vi "Main.vi"() -> ()   [LabVIEW 2011]
doc: "Use this template to build a simple state machine design pattern. Each state executes code and determines which state to transition to."
uses:
  controls/Data.ctl
  controls/State.ctl
panel:
  in  "Feeder Input":i16=1
  in  "Corridor Input":i16=2
  out "refnum out":refnum<k1>
  in  "Feeder Delay":u32=500
  in  "Corridor Delay":u32=500
  in  "Sample Delay":i32=50
  out "Data":T1
  out "Beam":u32
  in  "@Feeder":bool
  in  "Feeder Enable":bool
  in  "EoCo":bool
  in  "Exit":bool
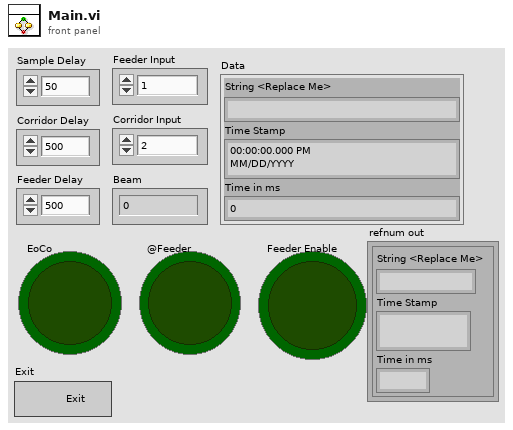
[diagram p1: front panel]
types:
  T1 = typedef "Data.ctl" = cluster{"String <Replace Me>":string, "Time Stamp":timestamp, "Time in ms":dbl}
  T2 = typedef "State.ctl" = enum16{"Initialize", "Refresh", "Wait for Event", "End of Corridor", "End of Corridor Delay", "Feed", "Feed Delay", "Exit"}
  T3 = enum16{"open", "replace", "create", "open or create", "replace or create", "replace or create with confirmation"}
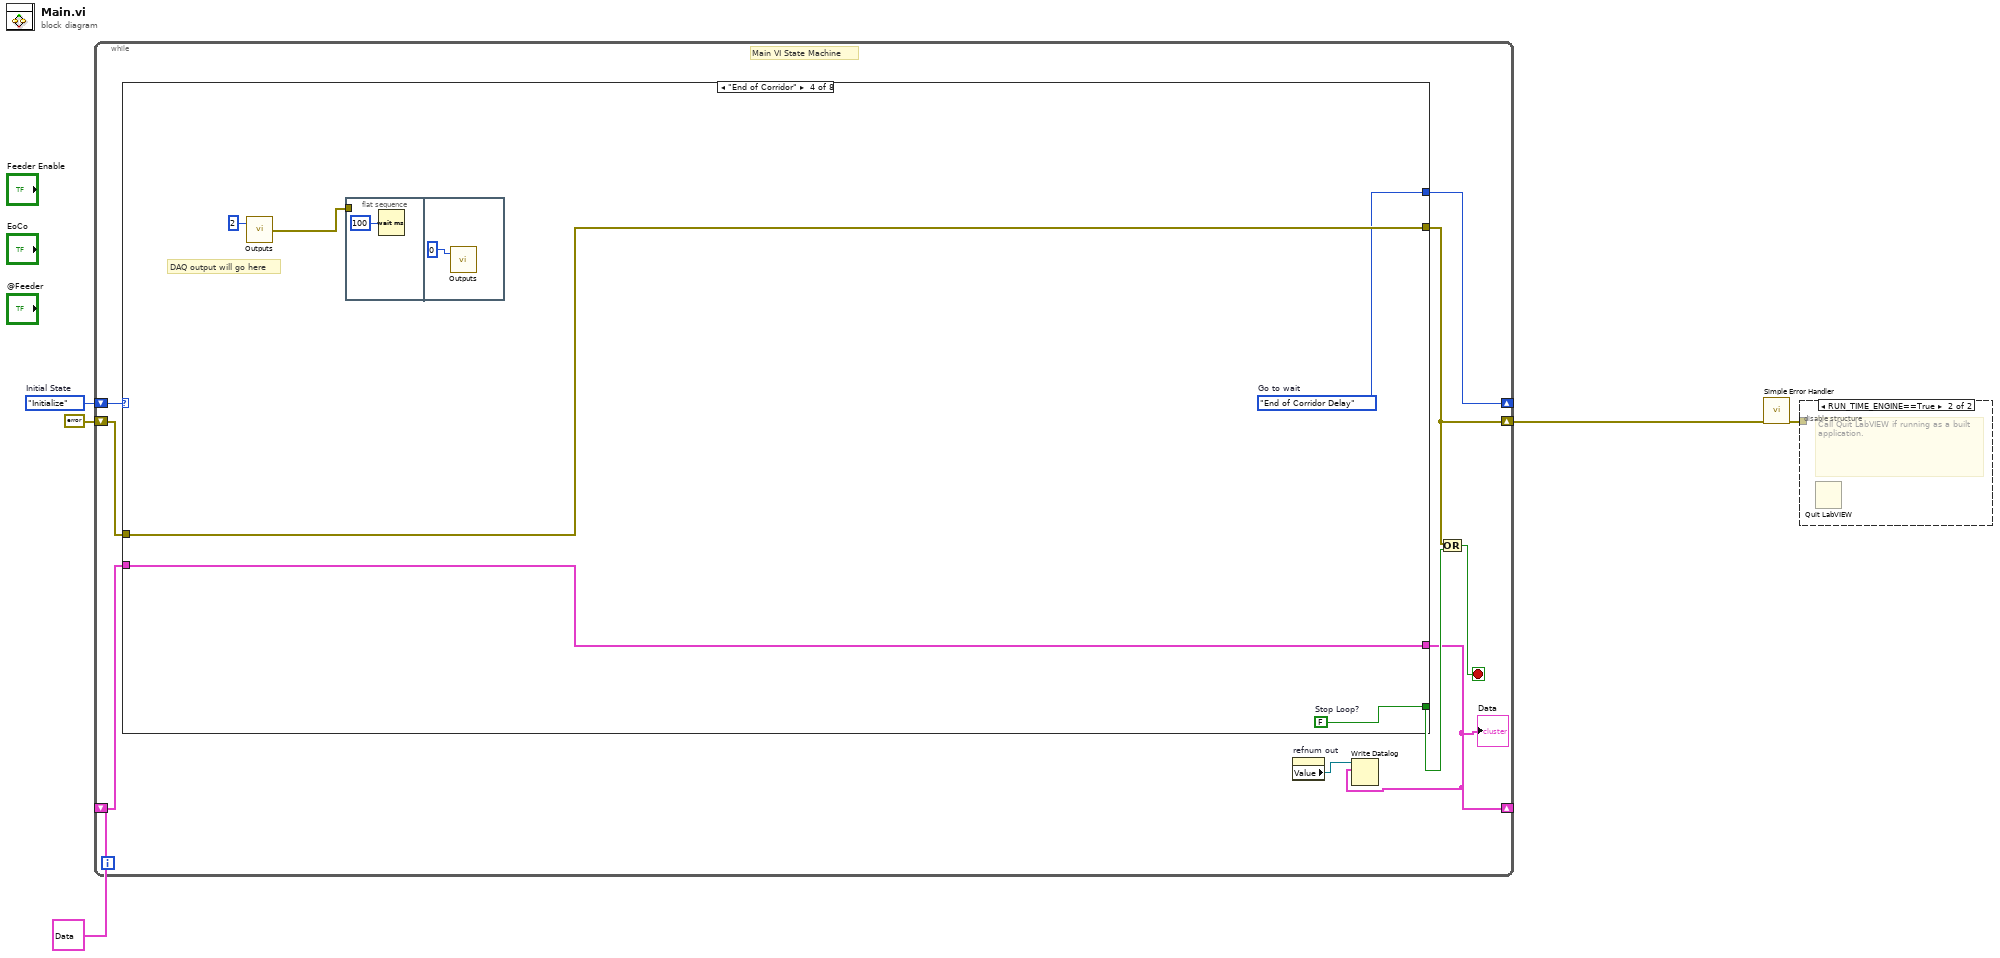
[diagram p0: block diagram]
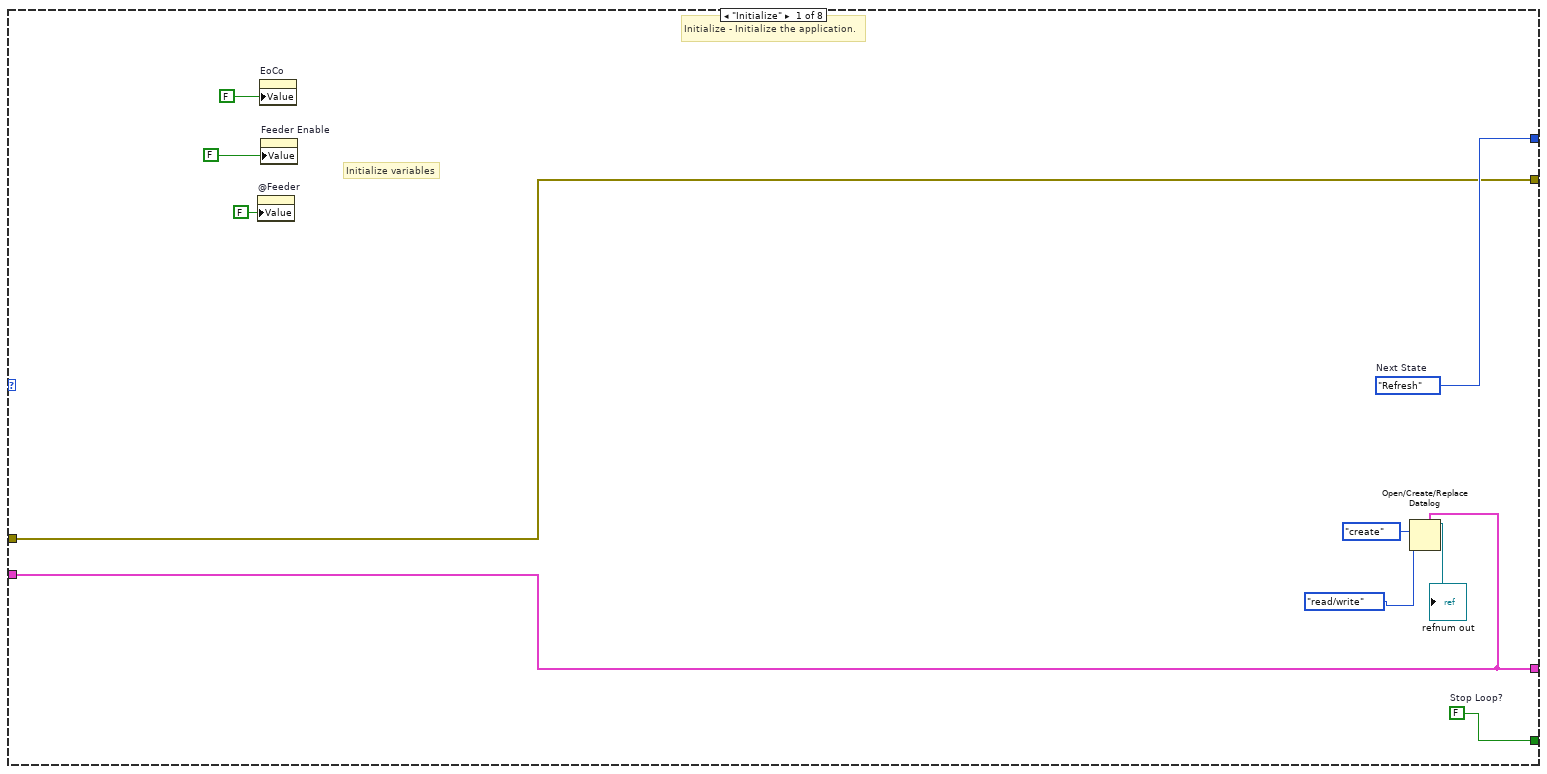
[diagram p3: hidden frame]
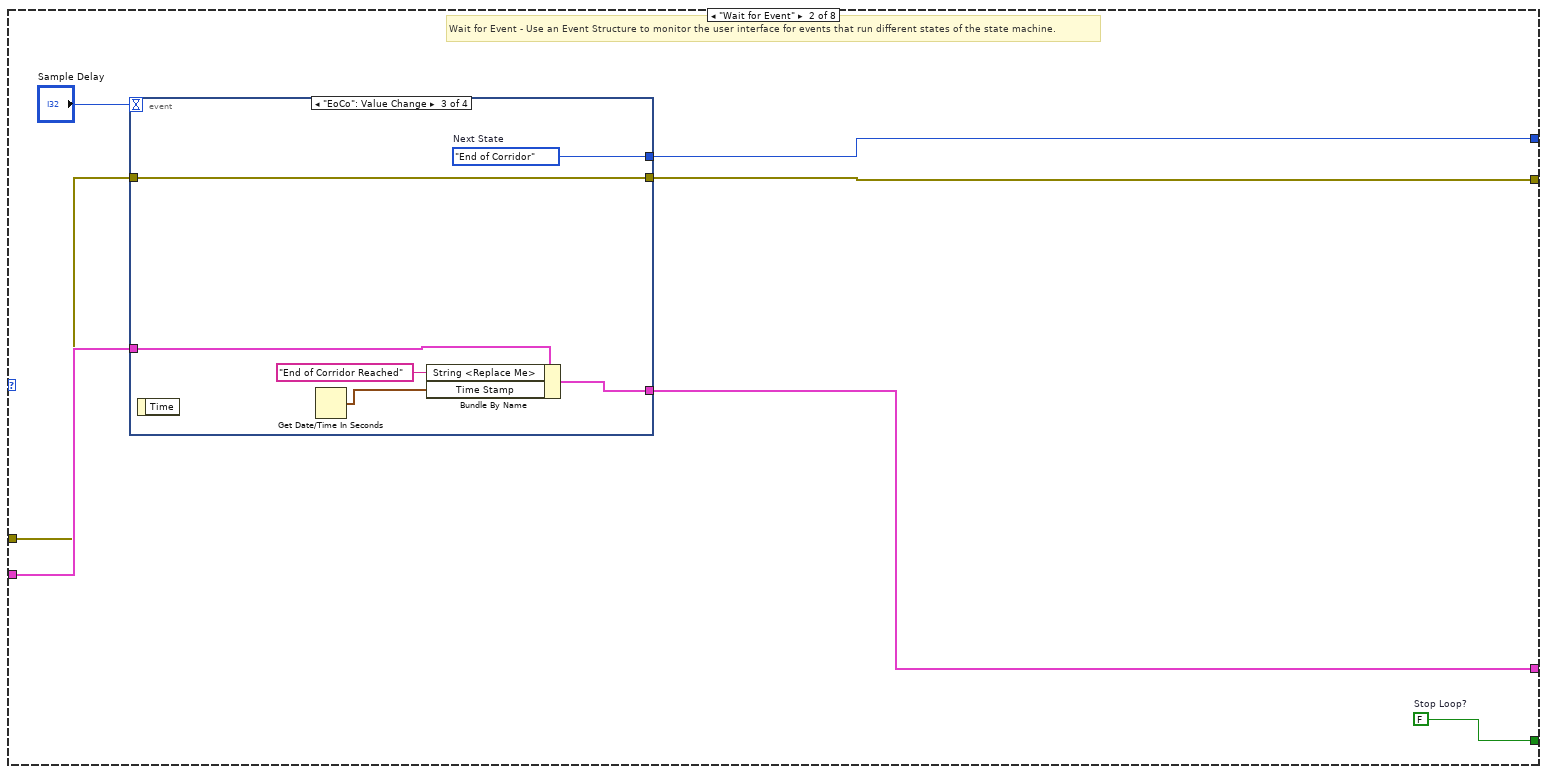
[diagram p4: hidden frame]
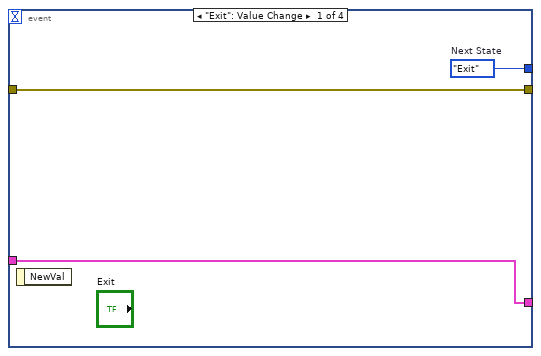
[diagram p5: hidden frame]
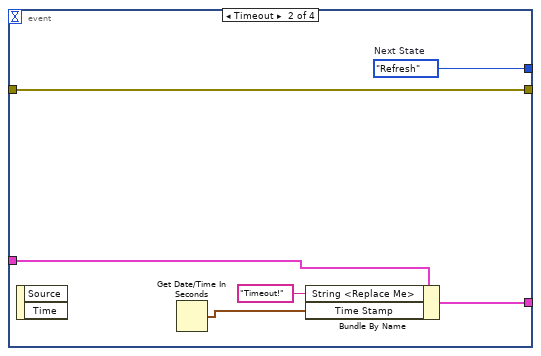
[diagram p6: hidden frame]
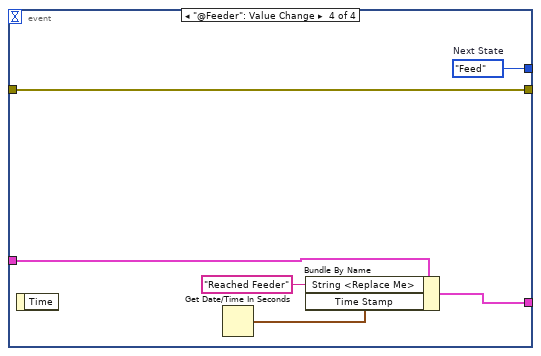
[diagram p7: hidden frame]
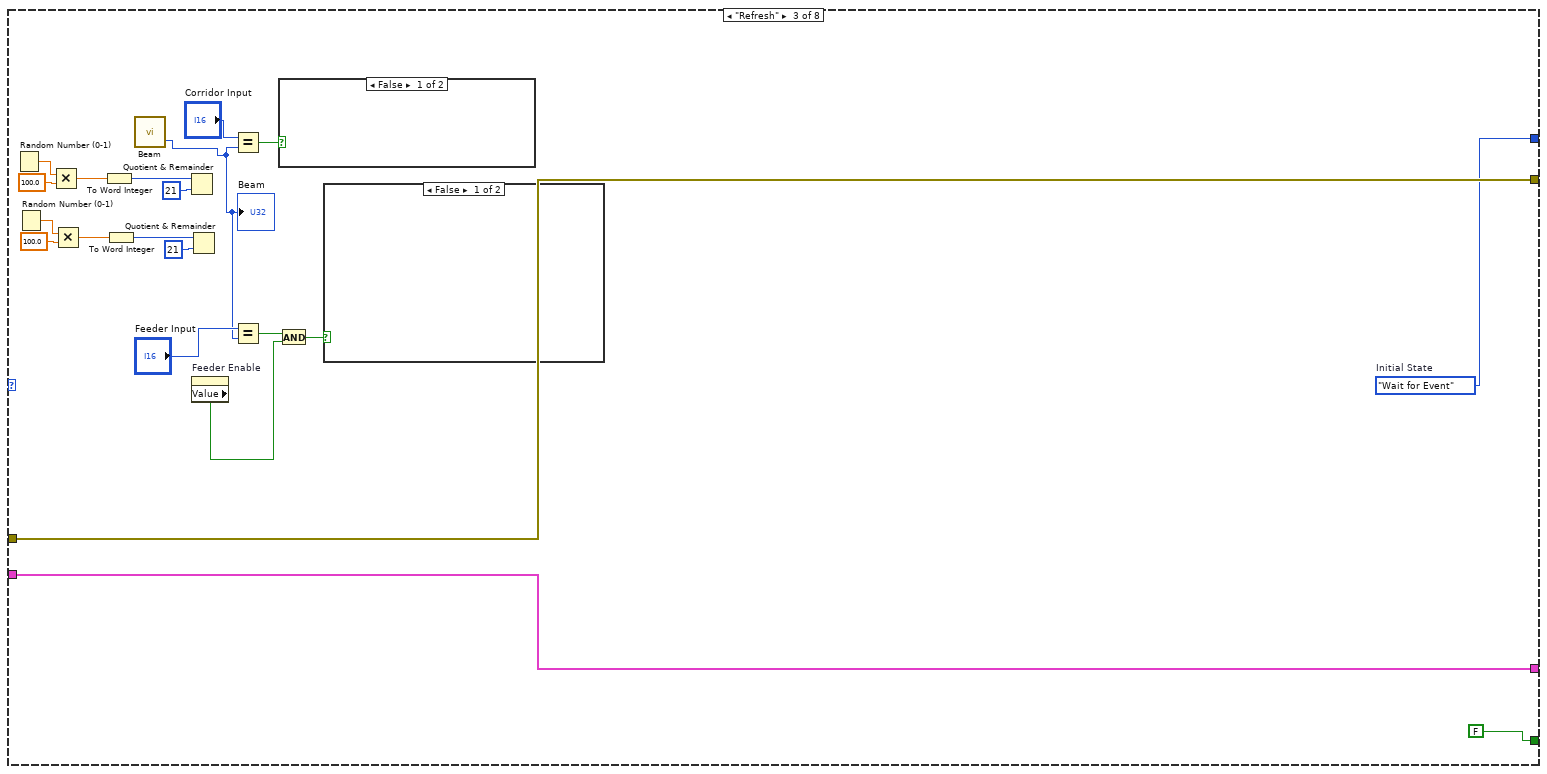
[diagram p8: hidden frame]
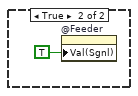
[diagram p9: hidden frame]
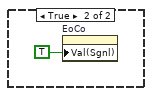
[diagram p10: hidden frame]
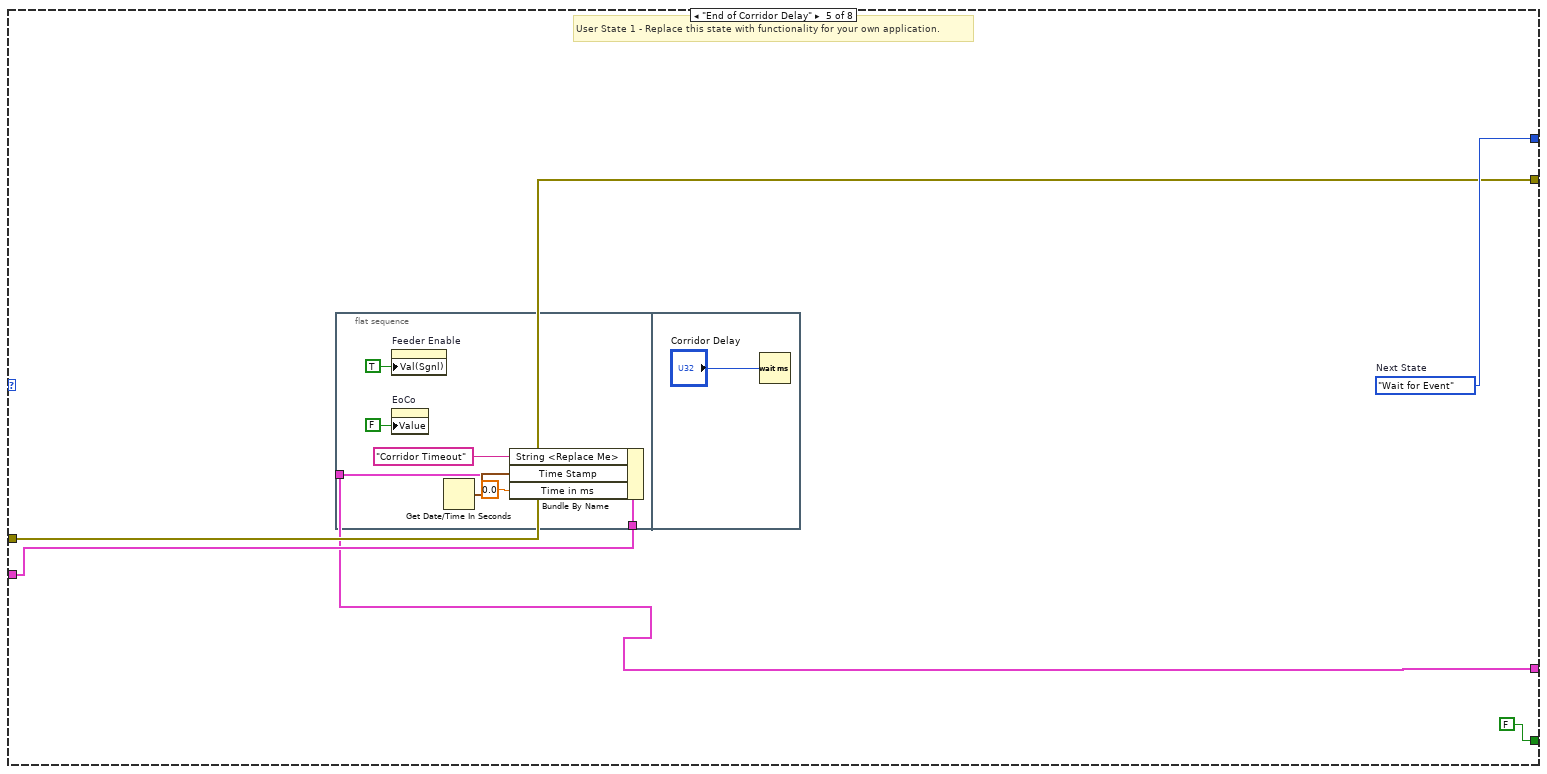
[diagram p11: hidden frame]
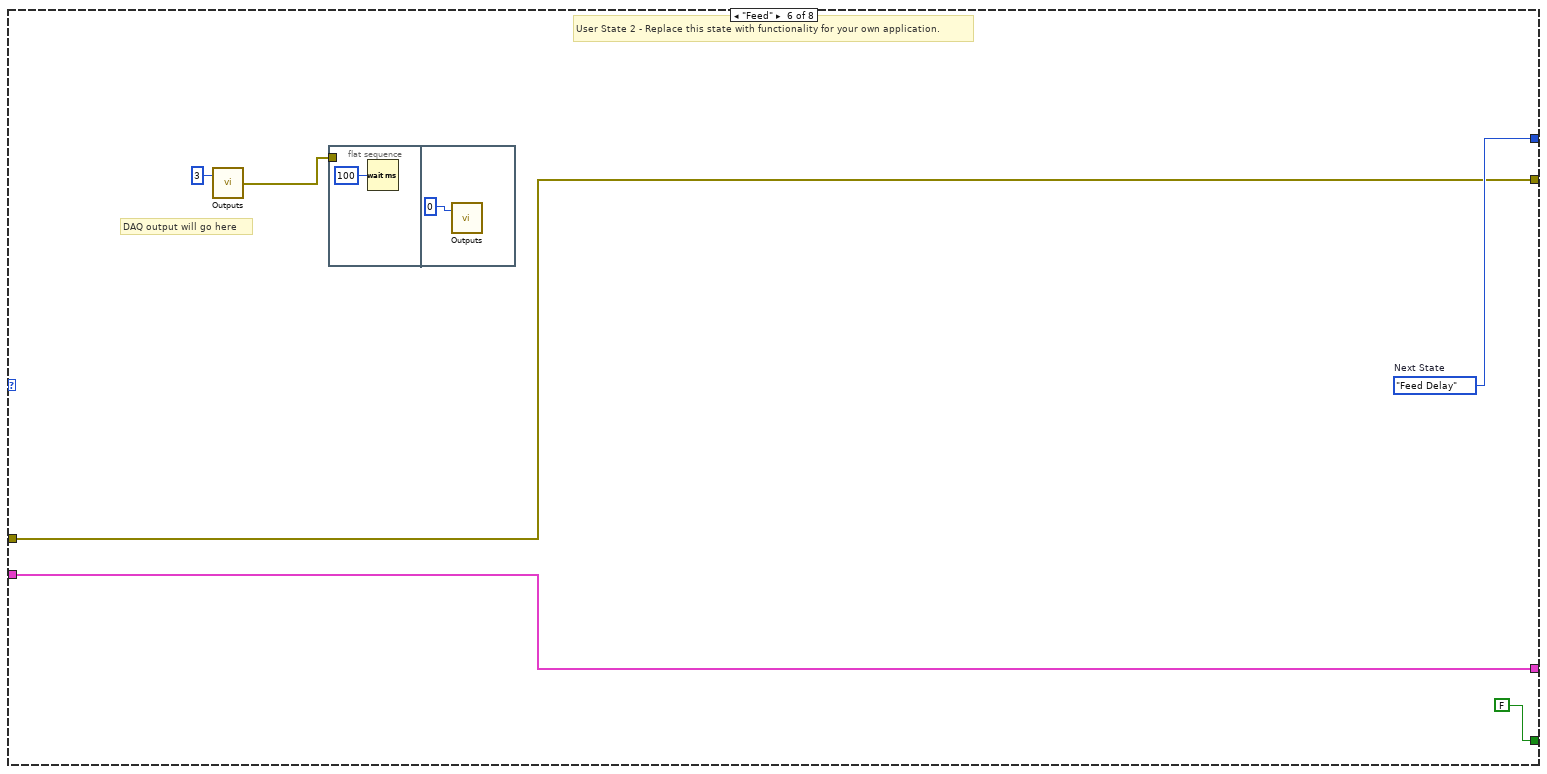
[diagram p12: hidden frame]
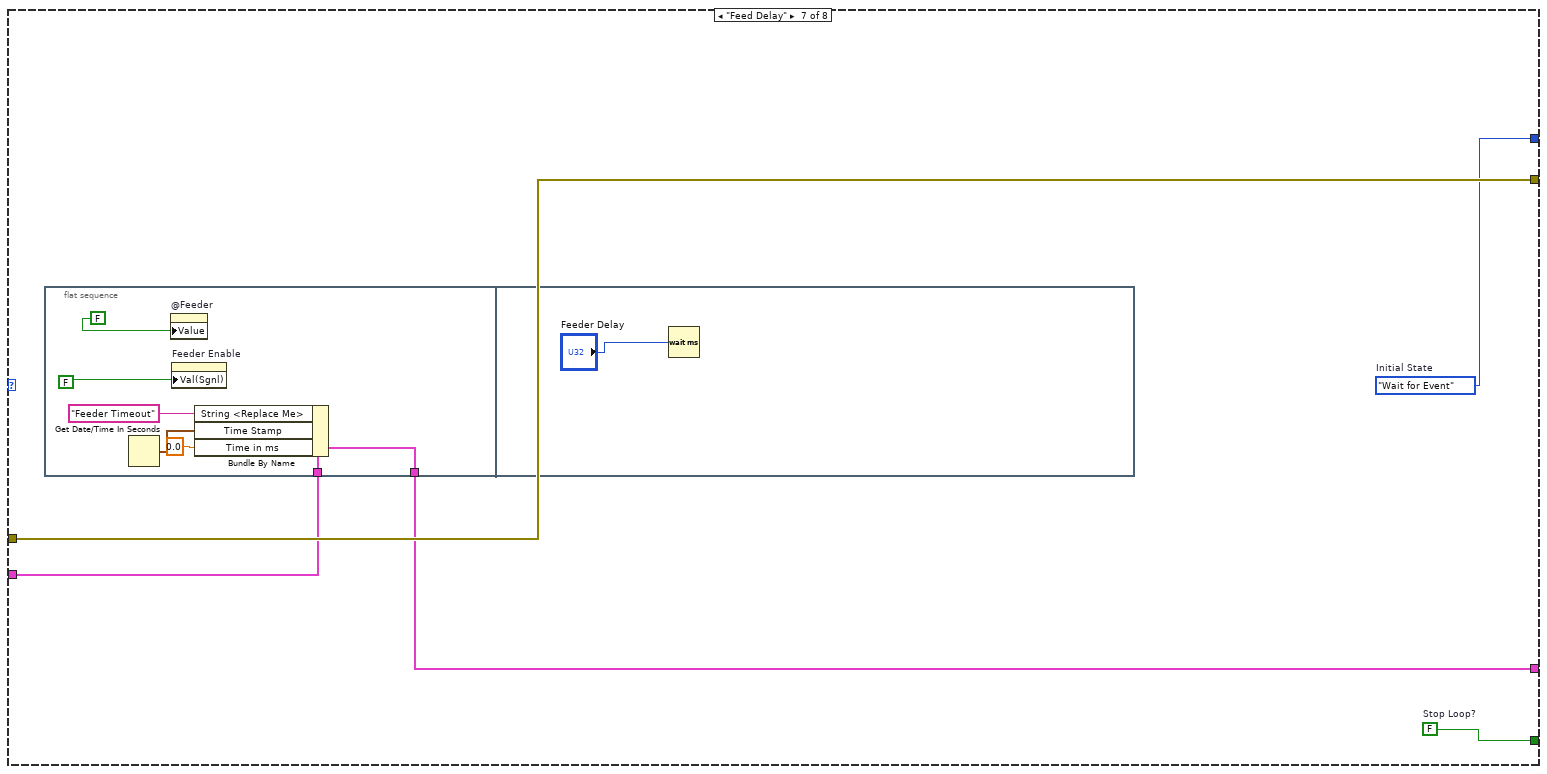
[diagram p13: hidden frame]
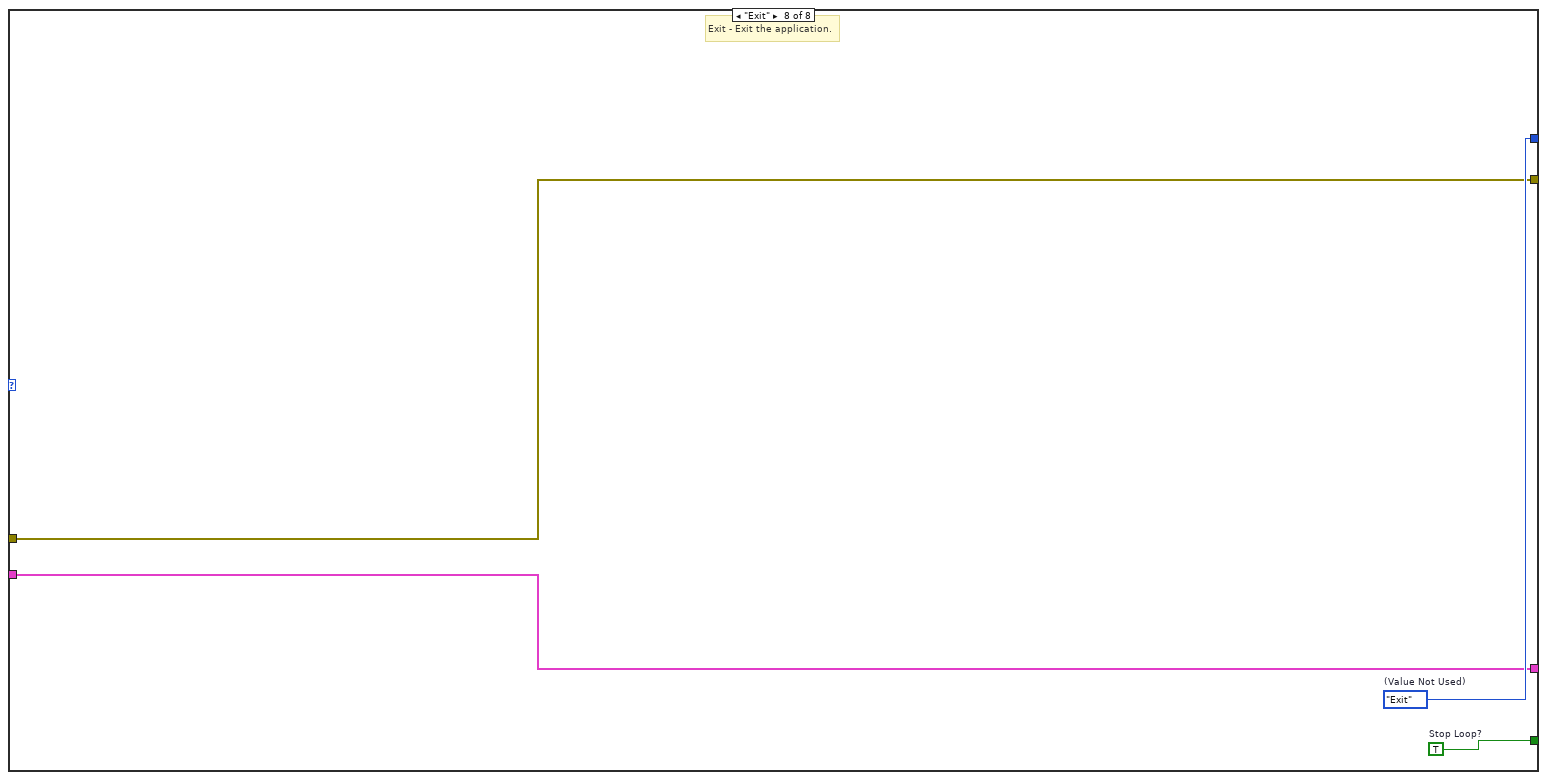
[diagram p14: hidden frame]
diagram:
  w5 = State."Initialize"  # Initial State
  n1 = while {
    shift-right: [w13] -> _
    shift-left: w5 -> [w14]
    shift-right: [w7] -> _
    shift-left: T1 {"String <Replace Me>"="", "Time Stamp"=timestamp(0 s since 1904-01-01), "Time in ms"=0.0} ("Data") -> [w12]
    shift-right: [w8] -> w2
    shift-left: errorcluster {"status"=FALSE, "code"=0, "source"=""} ("error constant") -> [w11]
    stop <- w9 stop-if-true
    # "Main VI State Machine"
    n2 = case shown="\"End of Corridor\"" w14 {
      tunnel: [w24 w31 w71 w79 w88 w102 w108 w121] -> w13
      tunnel: [w23 w30 FALSE ("Stop Loop?") w78 FALSE ("Stop Loop?") FALSE ("Stop Loop?") w107 w118] -> w10
      tunnel: w12 -> [w16 w29 w73 w81 w85 w100 w106 w120]
      tunnel: [w16 w28 w73 w81 w84 w100 w105 w120] -> w7
      tunnel: w11 -> [w22 w27 w72 w80 w86 w99 w109 w119]
      tunnel: [w22 w26 w72 w80 w86 w99 w109 w119] -> w8
      frame "Initialize" {
        w23 = FALSE  # Stop Loop?
        w24 = State."Refresh"  # Next State
        # "Initialize variables"
        # "Initialize - Initialize the application."
        n3 = property on="@Feeder" class="Bool (strict)"("Value"=FALSE ("@Feeder")) -> ()  [unwired: 2 in, 2 out]
        n4 = property on="EoCo" class="Bool (strict)"("Value"=FALSE ("Value (Signaling)")) -> ()  [unwired: 2 in, 2 out]
        n5 = property on="Feeder Enable" class="Bool (strict)"("Value"=FALSE) -> ()  [unwired: 2 in, 2 out]
        n6 = Open/Create/Replace Datalog(5:w16, 9:enum16{"read/write", "read-only", "write-only"}."read/write" ("access (0:read/write)"), 10:T3."create" ("operation (0:open)")) -> (3:→"refnum out":refnum<k1>)  [unwired: 3 in, 2 out]
      }
      frame "Wait for Event" {
        w30 = FALSE  # Stop Loop?
        # "Wait for Event - Use an Event Structure to monitor the user interface for events that run different states of the state machine."
        n7 = event shown="[2] \"EoCo\": Value Change" {
          selector: _ -> [_ _ _ _]
          dyn-events: _ -> [_ _ _ _]
          timeout: "Sample Delay" -> [_ _ _ _]
          tunnel: [w34 w39 w46 w52] -> w31
          tunnel: w29 -> [w33 w36 w45 w51]
          tunnel: [w33 w38 w44 w50] -> w28
          tunnel: w27 -> [w32 w40 w42 w48]
          tunnel: [w32 w40 w42 w48] -> w26
          event "Exit": Value Change {
            w34 = State."Exit"  # Next State
            n8 = event-data() -> ()  [unwired: 1 in, 1 out]
          }
          event Timeout {
            w39 = State."Refresh"  # Next State
            n9 = event-data() -> ()  [unwired: 1 in, 2 out]
            n10 = Get Date/Time In Seconds() -> (seconds since 1Jan1904=w35:timestamp)
            n11 = Bundle By Name(cluster=w36, "String <Replace Me>"="Timeout!", "Time Stamp"=w35) -> (w38:T1)
          }
          event "EoCo": Value Change {
            w46 = State."End of Corridor"  # Next State
            n12 = event-data() -> ()  [unwired: 1 in, 1 out]
            n13 = Get Date/Time In Seconds() -> (seconds since 1Jan1904=w41:timestamp)
            n14 = Bundle By Name(cluster=w45, "String <Replace Me>"="End of Corridor Reached" ("Running User State 1"), "Time Stamp"=w41) -> (w44:T1)
          }
          event "@Feeder": Value Change {
            w52 = State."Feed"  # Next State
            n15 = event-data() -> ()  [unwired: 1 in, 1 out]
            n16 = Get Date/Time In Seconds() -> (seconds since 1Jan1904=w47:timestamp)
            n17 = Bundle By Name(cluster=w51, "String <Replace Me>"="Reached Feeder" ("Running User State 2"), "Time Stamp"=w47) -> (w50:T1)
          }
        }
      }
      frame "Refresh" {
        w71 = State."Wait for Event"  # Initial State
        n18 = Random Number (0-1)() -> (number: 0 to 1=w59:dbl)
        n19 = Random Number (0-1)() -> (number: 0 to 1=w66:dbl)
        n20 = Multiply(x=w59, y=100.0) -> (x*y=w60:dbl)
        n21 = Multiply(x=w66, y=100.0) -> (x*y=w65:dbl)
        n22 = To Word Integer(number=w60) -> (16bit integer=w61:i16)
        n23 = To Word Integer(number=w65) -> (16bit integer=w68:i16)
        n24 = call "Beam.vi"() -> ("return type"=w53:i16)  [unwired: 1 in, 1 out]
        "Beam" <- w53
        n25 = Quotient & Remainder(x=w61, y=u32 21) -> ()  [unwired: 2 out]
        n26 = Quotient & Remainder(x=w68, y=i16 21) -> ()  [unwired: 2 out]
        n27 = property on="Feeder Enable" class="Bool (strict)"() -> ("Value"=w70:bool)  [unwired: 2 in, 2 out]
        n28 = Equal?(x="Corridor Input", y=w53) -> (x = y?=w62:bool)
        n29 = Equal?(x="Feeder Input", y=w53) -> (x = y?=w63:bool)
        n30 = case shown="False" w62 {
          frame False {
          }
          frame True {
            n31 = property on="EoCo" class="Bool (strict)"("Val(Sgnl)"=TRUE ("Value (Signaling)")) -> ()  [unwired: 2 in, 2 out]
          }
        }
        n32 = And(x=w63, y=w70) -> (x .and. y?=w64:bool)
        n33 = case shown="False" w64 {
          frame False {
          }
          frame True {
            n34 = property on="@Feeder" class="Bool (strict)"("Val(Sgnl)"=TRUE ("Value (Signaling)")) -> ()  [unwired: 2 in, 2 out]
          }
        }
      }
      frame "End of Corridor" {
        w78 = FALSE  # Stop Loop?
        w79 = State."End of Corridor Delay"  # Go to wait
        # "DAQ output will go here"
        n35 = call "Outputs.vi"("Value"=i16 2) -> ("error out"=w77:errorcluster)  [unwired: 1 in]
        n36 = flat-sequence {
          tunnel: w77 -> [_]
          frame #0 {
            n37 = Wait (ms)(milliseconds to wait=u32 100) -> ()  [unwired: 1 out]
          }
          frame #1 {
            n38 = call "Outputs.vi"("Value"=i16 0) -> ()  [unwired: 1 in, 1 out]
          }
        }
      }
      frame "End of Corridor Delay" {
        w88 = State."Wait for Event"  # Next State
        # "User State 1 - Replace this state with functionality for your own application."
        n39 = flat-sequence {
          tunnel: w85 -> [w90]
          tunnel: [w89] -> w84
          frame #0 {
            n40 = property on="Feeder Enable" class="Bool (strict)"("Val(Sgnl)"=TRUE ("Value (Signaling)")) -> ()  [unwired: 2 in, 2 out]
            n41 = property on="EoCo" class="Bool (strict)"("Value"=FALSE ("Value (Signaling)")) -> ()  [unwired: 2 in, 2 out]
            n42 = Get Date/Time In Seconds() -> (seconds since 1Jan1904=w92:timestamp)
            n43 = Bundle By Name(cluster=w90, "String <Replace Me>"="Corridor Timeout", "Time Stamp"=w92, "Time in ms"=0.0) -> (w89:T1)
          }
          frame #1 {
            n44 = Wait (ms)(milliseconds to wait="Corridor Delay") -> ()  [unwired: 1 out]
          }
        }
      }
      frame "Feed" {
        w102 = State."Feed Delay"  # Next State
        # "DAQ output will go here"
        # "User State 2 - Replace this state with functionality for your own application."
        n45 = call "Outputs.vi"("Value"=i16 3) -> ("error out"=w98:errorcluster)  [unwired: 1 in]
        n46 = flat-sequence {
          tunnel: w98 -> [_]
          frame #0 {
            n47 = Wait (ms)(milliseconds to wait=u32 100) -> ()  [unwired: 1 out]
          }
          frame #1 {
            n48 = call "Outputs.vi"("Value"=i16 0) -> ()  [unwired: 1 in, 1 out]
          }
        }
      }
      frame "Feed Delay" {
        w107 = FALSE  # Stop Loop?
        w108 = State."Wait for Event"  # Initial State
        n49 = flat-sequence {
          tunnel: w106 -> [w111]
          tunnel: [w110] -> w105
          frame #0 {
            n50 = Get Date/Time In Seconds() -> (seconds since 1Jan1904=w113:timestamp)
            n51 = property on="@Feeder" class="Bool (strict)"("Value"=FALSE ("@Feeder")) -> ()  [unwired: 2 in, 2 out]
            n52 = property on="Feeder Enable" class="Bool (strict)"("Val(Sgnl)"=FALSE ("Value (Signaling)")) -> ()  [unwired: 2 in, 2 out]
            n53 = Bundle By Name(cluster=w111, "String <Replace Me>"="Feeder Timeout", "Time Stamp"=w113, "Time in ms"=0.0) -> (w110:T1)
          }
          frame #1 {
            n54 = Wait (ms)(milliseconds to wait="Feeder Delay") -> ()  [unwired: 1 out]
          }
        }
      }
      frame "Exit" {
        w118 = TRUE  # Stop Loop?
        w121 = State."Exit"  # (Value Not Used)
        # "Exit - Exit the application."
      }
    }
    "Data" <- w7
    n55 = property on="refnum out" class="TypRef (strict)"() -> ("Value"=w6:refnum<k1>)  [unwired: 2 in, 2 out]
    n56 = Write Datalog(6:w7, 7:w6) -> ()  [unwired: 1 in, 2 out]
    n57 = Or(x=w8, y=w10) -> (x .or. y?=w9:bool)
  }
  n58 = call <vilib>:"Simple Error Handler.vi"("error in (no error)"=w2) -> ("error out"=w1:errorcluster)  [unwired: 4 in, 4 out]
  n59 = disable-structure shown="RUN_TIME_ENGINE==True" {
    disable-tunnel: w1 -> [_ _]
    frame condition #0 (active) {
    }
    frame condition #1 {
      # "Call Quit LabVIEW if running as a built application."
      n60 = Quit LabVIEW() -> ()  [unwired: 1 in]
    }
  }
